vi "Test state machien.vi"() -> ()   [LabVIEW 2019]
uses:
  Gilson cmds.ctl
panel:
  out "appended array":bool[](array[boolean])
  out "Receive string":string
  out "error out":errorcluster
  in  "ID (1)":u8=1
  in  "VISA resource name":refnum<visa-resource-name>="COM1"
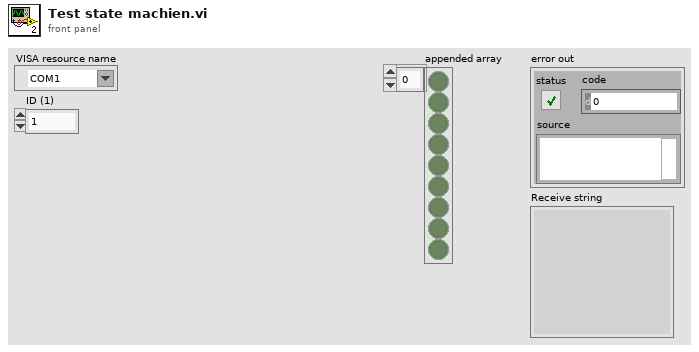
[diagram p1: front panel]
types:
  T1 = typedef "Gilson cmds.ctl" = enum16{"Initialize Port", "Immediate", "Buffered", "Connect", "Close Port"}
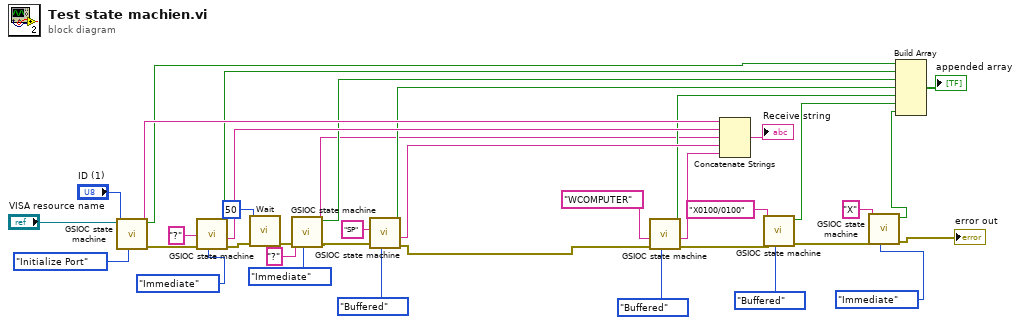
[diagram p0: block diagram]
diagram:
  n1 = call "GSIOC state machine.vi"("GSIOC cmd"=Gilson_cmds."Initialize Port", "ID (1)"="ID (1)", "VISA resource name"="VISA resource name") -> ("error out"=w35:errorcluster, "Receive string"=w28:string, "Connected"=w15:bool)  [unwired: 5 in, 1 out]
  n2 = call "GSIOC state machine.vi"("GSIOC cmd"=Gilson_cmds."Immediate", "error in (no error)"=w35, "Command"="?") -> ("error out"=w8:errorcluster, "Receive string"=w26:string, "Connected"=w14:bool)  [unwired: 5 in, 1 out]
  n3 = call "Wait.vi"("error in"=w8, "milliseconds to wait"=u32 50) -> ("error out"=w6:errorcluster)  [unwired: 9 in]
  n4 = call "GSIOC state machine.vi"("GSIOC cmd"=Gilson_cmds."Immediate", "error in (no error)"=w6, "Command"="?") -> ("error out"=w5:errorcluster, "Receive string"=w1:string, "Connected"=w3:bool)  [unwired: 5 in, 1 out]
  n5 = call "GSIOC state machine.vi"("GSIOC cmd"=Gilson_cmds."Buffered", "error in (no error)"=w5, "Command"="SP") -> ("error out"=w16:errorcluster, "Receive string"=w25:string, "Connected"=w13:bool)  [unwired: 5 in, 1 out]
  n6 = call "GSIOC state machine.vi"("GSIOC cmd"=Gilson_cmds."Buffered", "error in (no error)"=w16, "Command"="WCOMPUTER") -> ("error out"=w20:errorcluster, "Receive string"=w24:string, "Connected"=w12:bool)  [unwired: 5 in, 1 out]
  n7 = Concatenate Strings(w28, w26, w1, w25, w24) -> (→"Receive string":string)
  n8 = call "GSIOC state machine.vi"("GSIOC cmd"=Gilson_cmds."Buffered", "error in (no error)"=w20, "Command"="X0100/0100") -> ("error out"=w19:errorcluster, "Connected"=w11:bool)  [unwired: 5 in, 2 out]
  n9 = call "GSIOC state machine.vi"("GSIOC cmd"=Gilson_cmds."Immediate", "error in (no error)"=w19, "Command"="X") -> ("error out"=→"error out":errorcluster, "Connected"=w10:bool)  [unwired: 5 in, 2 out]
  n10 = Build Array(w15, w14, w3, w13, w12, w11, w10) -> (→"appended array":bool[])
